vi "KE622x -- Set Filter Params.vi"(0 "Resource In":refnum<visa-resource-name>, 1 "Check For SCPI Errors? (T)":bool=TRUE, 7 "Filter Params In":T1={"Filter Enabled?"=FALSE, "Filter Type"=enum."Moving Ave", "Filter Length"=10, "Filter Window (%)"=0.0} {"Filter Window (%)" min=0.0 max=10.0 step=0.01 format="%.2f"; "Filter Length" min=2 max=300}, 11 "error in (no error)":errorcluster, 12 "Read Back Set Values? (T)":bool=TRUE) -> (4 "Resource Out (dupl)":refnum<visa-resource-name>, 8 "Filter Params Out":T1={"Filter Enabled?"=FALSE, "Filter Type"=enum."Moving Ave", "Filter Length"=10, "Filter Window (%)"=0.0} {"Filter Window (%)" min=0.0 max=10.0 step=0.01 format="%.2f"; "Filter Length" min=2 max=300}, 15 "error out":errorcluster)   [LabVIEW 2020, in "Keithley 622x.lvlib"]
doc: "Sets the parameters of the digital filter in the instrument, and also whether or not the filter is enabled. Note that since the 622x instrument doesn't really make any measurements, use of the digital implies that the 622x is being used in conjunction with a 2182/2182A nano-voltmeter."
uses:
  Keithley 622x.lvlib
  <instrlib>/Keithley 622x LV 2009/Configure/Sense/Typedefs/KE622x -- Filter Params.ctl
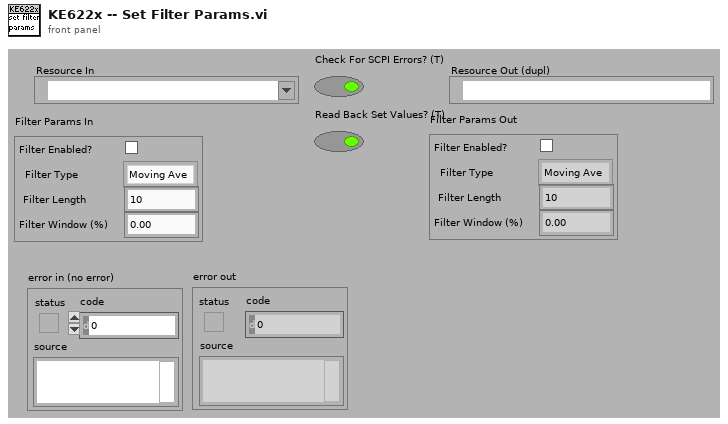
[diagram p1: front panel]
types:
  T1 = typedef "Keithley 622x.lvlib/KE622x -- Filter Params.ctl" = cluster{"Filter Enabled?":bool, "Filter Type":enum16{"Moving Ave", "Repeat Ave"}, "Filter Length":u32, "Filter Window (%)":dbl}
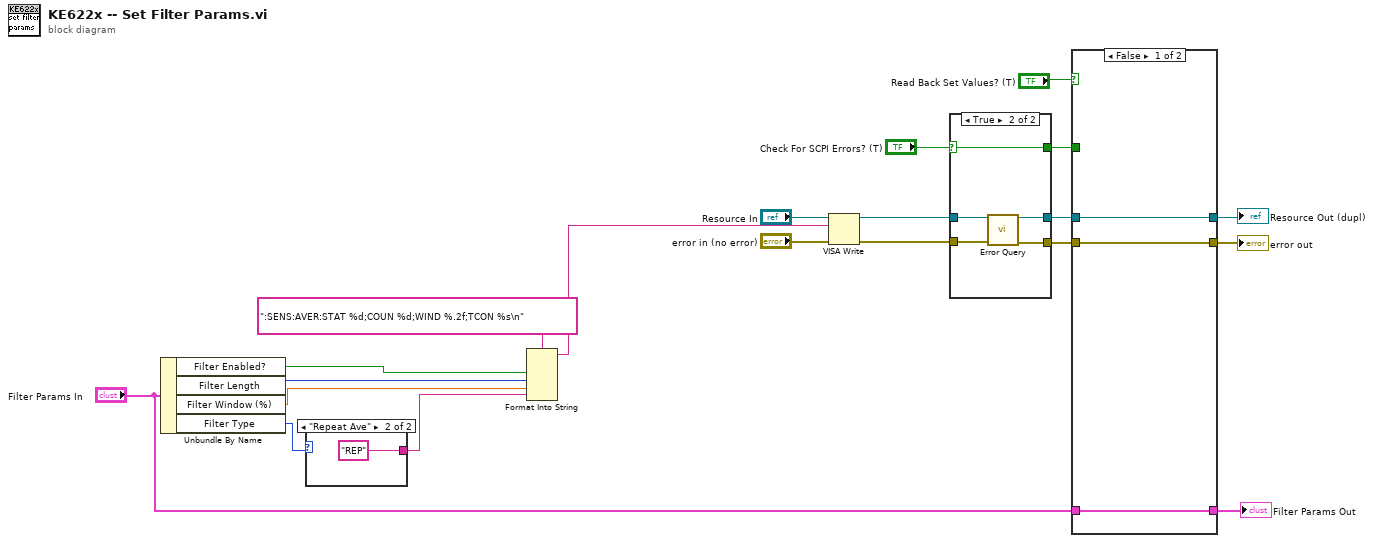
[diagram p0: block diagram]
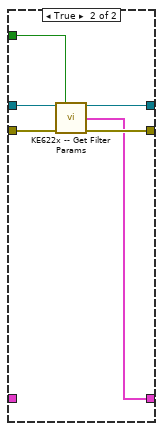
[diagram p2: hidden frame]
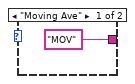
[diagram p3: hidden frame]
diagram:
  n1 = Unbundle By Name("Filter Params In") -> ("Filter Enabled?"=w14:bool, "Filter Length"=w12:u32, "Filter Window (%)"=w11:dbl, "Filter Type"=w10:enum16{"Moving Ave", "Repeat Ave"})
  n2 = case shown="\"Repeat Ave\"" w10 {
    tunnel: ["MOV" "REP"] -> w9
    frame "Moving Ave" {
    }
    frame "Repeat Ave" {
    }
  }
  n3 = Format Into String(format string=":SENS:AVER:STAT %d;COUN %d;WIND %.2f;TCON %s\n", w14, w12, w11, w9) -> (resulting string=w13:string)  [unwired: 2 in, 1 out]
  n4 = VISA Write(VISA resource name="Resource In", write buffer=w13, error in (no error)="error in (no error)") -> (VISA resource name out=w17:refnum<visa-resource-name>, error out=w16:errorcluster)  [unwired: 1 out]
  n5 = case shown="True" "Check For SCPI Errors? (T)" {
    selector: "Check For SCPI Errors? (T)" -> [w23 w26]
    tunnel: w17 -> [w25 w30]
    tunnel: w16 -> [w24 w29]
    tunnel: [w24 w28] -> w6
    tunnel: [w25 w27] -> w7
    tunnel: [w23 w26] -> w5
    frame False {
    }
    frame True {
      n6 = call "Error Query.vi"("VISA Resource In"=w30, "error in (no error)"=w29) -> ("VISA Resource Out (dupl)"=w27:refnum<visa-resource-name>, "error out"=w28:errorcluster)  [unwired: 10 in, 2 out]
    }
  }
  n7 = case shown="False" "Read Back Set Values? (T)" {
    tunnel: w7 -> [w32 w39]
    tunnel: w6 -> [w31 w38]
    tunnel: w5 -> [_ w37]
    tunnel: [w32 w36] -> w4
    tunnel: [w31 w35] -> w3
    tunnel: "Filter Params In" -> [w33 _]
    tunnel: [w33 w34] -> w1
    frame False {
    }
    frame True {
      n8 = call "KE622x -- Get Filter Params.vi"("Resource In"=w39, "Check For SCPI Errors? (T)"=w37, "error in (no error)"=w38) -> ("Resource Out (dupl)"=w36:refnum<visa-resource-name>, "Filter Params"=w34:T1, "error out"=w35:errorcluster)  [unwired: 10 in]
    }
  }
  "Resource Out (dupl)" <- w4
  "error out" <- w3
  "Filter Params Out" <- w1
